vi "libssh2_knownhost_get - no previous - returns first host.vi"() -> ()   [LabVIEW 2017, in "unit_tests.lvlib"]
uses:
  unit_tests.lvlib
  libssh2/libssh2_init_default.vi
  libssh2/libssh2_session_init_ex.vi
  libssh2/libssh2.lvlib
  <vilib>/PNR/Transparent Assertions/Transparent Assertions/Transparent Assertions.lvlib
panel:
  out "error out":errorcluster
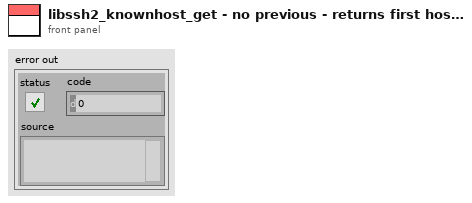
[diagram p1: front panel]
types:
  T1 = typedef "libssh2.lvlib/Session Refnum.ctl" = refnum<k1>
  T2 = typedef "libssh2.lvlib/Host Key Database Refnum.ctl" = refnum<k1>
  T3 = typedef "libssh2.lvlib/Host Key Refnum.ctl" = refnum<k1>
  T4 = typedef "libssh2.lvlib/libssh2_knownhost.ctl" = cluster{"magic":u32, "node":u64, "name":string, "key":string, "typemask":i32}
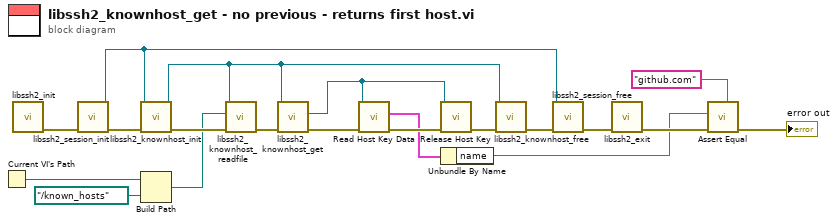
[diagram p0: block diagram]
diagram:
  n1 = Current VI's Path() -> (path=w11:path)
  n2 = call-poly "libssh2_init.vi"() -> ("error out"=w19:errorcluster)  [unwired: 11 in]
  n3 = call "libssh2_session_init.vi"("error in (no error)"=w19) -> ("error out"=w18:errorcluster, "session"=w15:T1)  [unwired: 9 in]
  n4 = call "libssh2_knownhost_init.vi"("error in (no error)"=w18, "session"=w15) -> ("error out"=w13:errorcluster, "host key database"=w8:T2)  [unwired: 8 in]
  n5 = Build Path(base path=w11, name or relative path=path "../known_hosts" ("filename")) -> (appended path=w9:path)
  n6 = call "libssh2_knownhost_readfile.vi"("error in (no error)"=w13, "filename"=w9, "host key database"=w8) -> ("error out"=w12:errorcluster)  [unwired: 7 in, 1 out]
  n7 = call "libssh2_knownhost_get.vi"("error in (no error)"=w12, "host key database"=w8) -> ("error out"=w6:errorcluster, "host key"=w4:T3)  [unwired: 7 in, 1 out]
  n8 = call "Read Host Key Data.vi"("error in (no error)"=w6, "host key"=w4) -> ("error out"=w5:errorcluster, "host key data"=w3:T4)  [unwired: 8 in]
  n9 = call "Release Host Key.vi"("error in (no error)"=w5, "host key"=w4) -> ("error out"=w7:errorcluster)  [unwired: 9 in]
  n10 = Unbundle By Name(w3) -> ("name"=w2:string)
  n11 = call "libssh2_knownhost_free.vi"("error in (no error)"=w7, "host key database"=w8) -> ("error out"=w14:errorcluster)  [unwired: 9 in]
  n12 = call "libssh2_session_free.vi"("error in (no error)"=w14, "session"=w15) -> ("error out"=w17:errorcluster)  [unwired: 9 in]
  n13 = call "libssh2_exit.vi"("error in (no error)"=w17) -> ("error out"=w16:errorcluster)  [unwired: 10 in]
  n14 = call <vilib>:"Assert Equal.vi"("Expected"="github.com" ("key"), "error in (no error)"=w16, "Actual"=w2) -> ("error out"=→"error out":errorcluster)  [unwired: 8 in]
